vi "n set matrix list.vi"(7 "mij":dbl, 8 "error in (no error)":errorcluster, 9 "j":u16, 10 "i":u16, 11 "n":u16) -> (0 "error out":errorcluster)   [LabVIEW 2015, in "SCANalone4x64.lvlib"]
doc: "__declspec(dllimport) void __stdcall n_set_matrix_list(unsigned short n, unsigned short i, unsigned short j, double mij);"
uses:
  <userlib>/SCANalone4x64/SCANalone4x64.lvlib
  <userlib>/SCANalone4x64/SCANalone4x64.dll
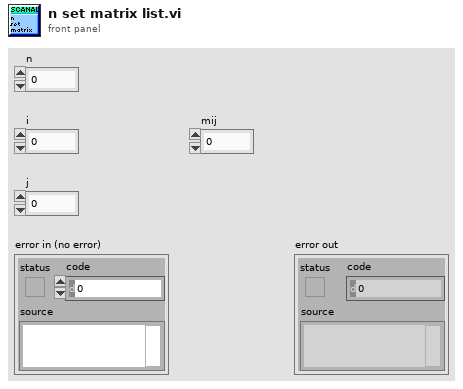
[diagram p1: front panel]
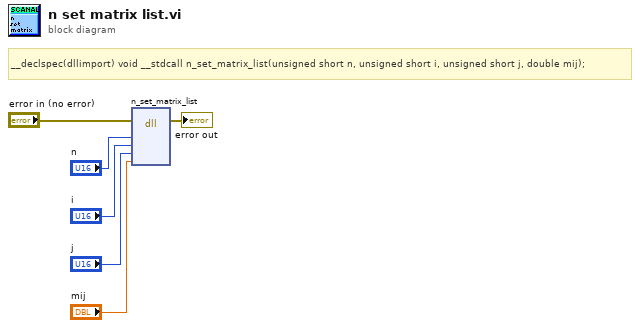
[diagram p0: block diagram]
diagram:
  # "__declspec(dllimport) void __stdcall n_set_matrix_list(unsigned short n, unsigned short i, unsigned short j, double mij);"
  n1 = dll-call lib="C:/Program Files/National Instruments/LabVIEW 2015/user.lib/SCANalone4x64/SCANalone4x64.*" fn="n_set_matrix_list"(error in="error in (no error)", "n"="n", "i"="i", "j"="j", "mij"="mij") -> (error out=→"error out":errorcluster)  [unwired: 7 in, 1 out]
